vi "DecodeAvs47bReading.vi"(8 "LV ERROR IN":errorcluster, 10 "RXSTR":string="000000111001000000011000000000001100000010000000", 11 "CONFIGURATION CLUSTER":T1) -> (0 "LV ERROR OUT":errorcluster, 1 "ADC":i32, 2 "RESISTANCE":sgl format="%^#_6e", 3 "UNMODIFIED CONFIGURATION CLUSTER":T1, 4 "RESISTANCE STRING":string="0 ohm", 5 "ADC OVERRANGE":bool)   [LabVIEW 2023]
doc: "Used by ReadAvs47b.vi \nResistance given as real number"
panel:
  out "4 empty bits (hidden)":u16
  # "DecodeAvs47Reading.vi"
  # "(input to this VI)"
  # "(outputs)"
  # "(ohms)"
  # "Extracts the A/D conversion result from the Picobus return string RXSTR and \nexpresses the measured resistance as a floating point number. Also a string\nrepresentation with unit is provided for display purposes."
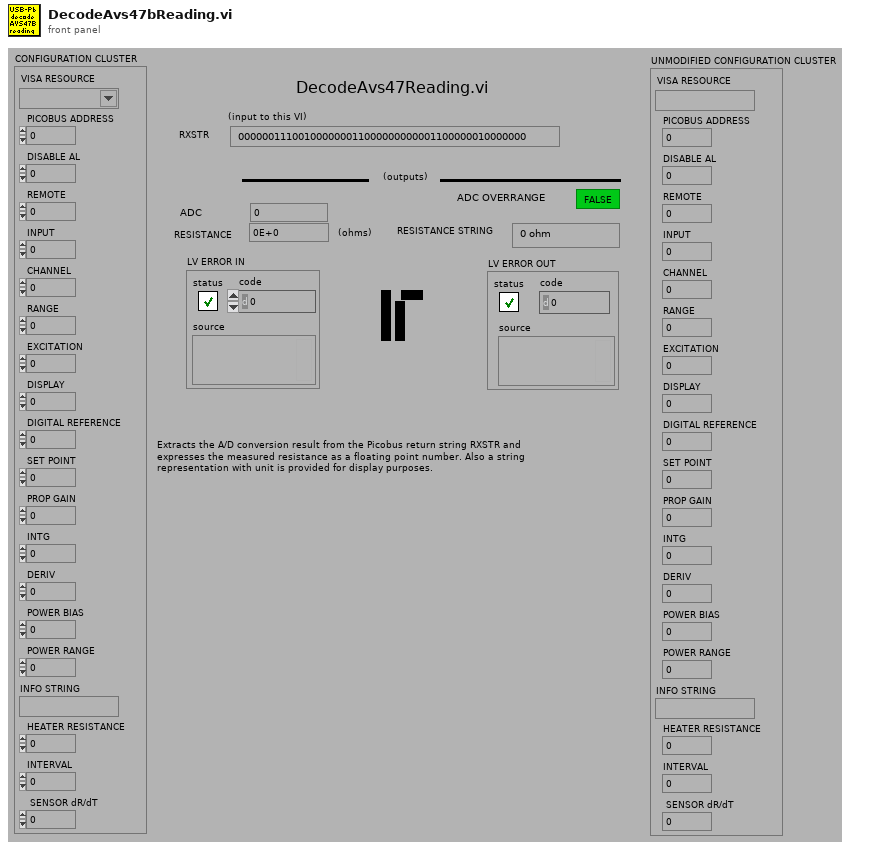
[diagram p1: front panel]
types:
  T1 = cluster{"VISA RESOURCE":refnum<visa-resource-name>, "PICOBUS ADDRESS":u8, "DISABLE AL":u8, "REMOTE":u8, "INPUT":u8, "CHANNEL":u8, "RANGE":u8, "EXCITATION":u8, "DISPLAY":u8, "DIGITAL REFERENCE":u16, "SET POINT":dbl, "PROP GAIN":u8, "INTG":u8, "DERIV":u8, "POWER BIAS":u8, "POWER RANGE":u8, "INFO STRING":string, "HEATER RESISTANCE":dbl, "INTERVAL":u8, " SENSOR dR/dT":u8}
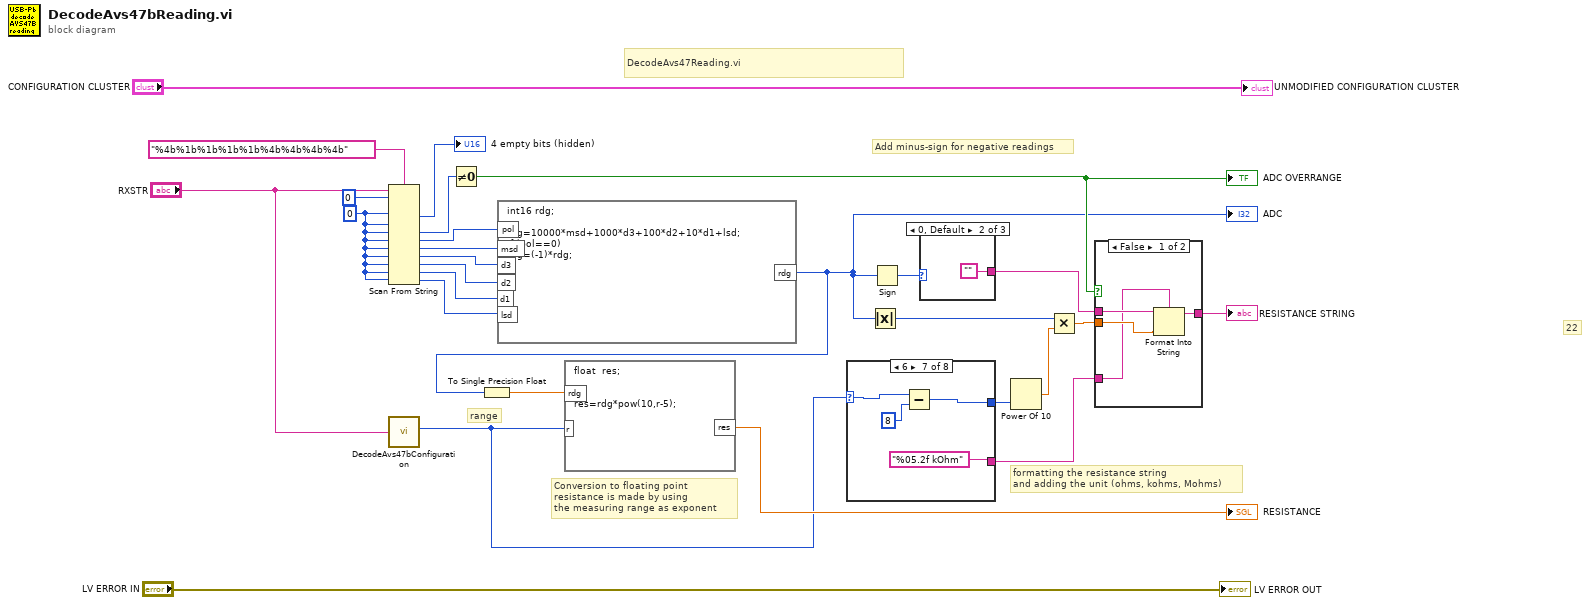
[diagram p0: block diagram]
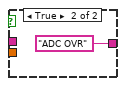
[diagram p2: hidden frame]
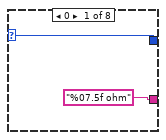
[diagram p3: hidden frame]
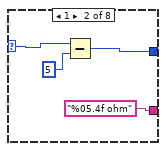
[diagram p4: hidden frame]
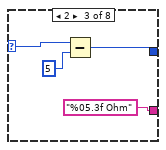
[diagram p5: hidden frame]
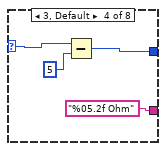
[diagram p6: hidden frame]
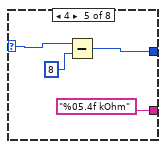
[diagram p7: hidden frame]
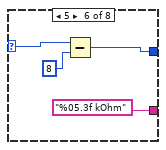
[diagram p8: hidden frame]
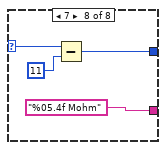
[diagram p9: hidden frame]
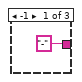
[diagram p10: hidden frame]
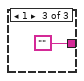
[diagram p11: hidden frame]
diagram:
  w24 = u16 0
  # "22"
  # "Add minus-sign for negative readings"
  # "formatting the resistance string\nand adding the unit (ohms, kohms, Mohms)"
  # "Conversion to floating point\nresistance is made by using \nthe measuring range as exponent"
  # "BCD-to-decimal\nconversion. Result\nis a 4 1/2 digit integer"
  # "range"
  # "DecodeAvs47Reading.vi"
  n1 = Scan From String(format string="%4b%1b%1b%1b%1b%4b%4b%4b%4b", input string="RXSTR", initial scan location=u16 0, default 1=w24, default 2=w24, default 3=w24, default 4=w24, default 5=w24, default 6=w24, default 7=w24, default 8=w24, default 9=w24) -> (output 1=→"4 empty bits (hidden)":u16, output 3=w14:u16, output 4=w18:u16, output 5=w23:u16, output 6=w22:u16, output 7=w21:u16, output 8=w20:u16, output 9=w19:u16)  [unwired: 2 in, 3 out]
  n2 = call "DecodeAvs47bConfiguration.vi"("RXSTR"="RXSTR") -> ("RANGE OUT"=w3:u16)  [unwired: 5 in, 4 out]
  n3 = Not Equal To 0?(x=w14) -> (x != 0?=w4:bool)
  "ADC OVERRANGE" <- w4
  n4 = formula code="int16 rdg;\n\nrdg=10000*msd+1000*d3+100*d2+10*d1+lsd;\nif (pol==0)\nrdg=(-1)*rdg;"("msd"=w23, "d3"=w22, "d2"=w21, "d1"=w20, "lsd"=w19, "pol"=w18) -> ("rdg"=w2:i16)
  "ADC" <- w2
  n5 = To Single Precision Float(number=w2) -> (single precision float=w16:sgl)
  n6 = formula code="float  res;\n\n\nres=rdg*pow(10,r-5);"("r"=w3, "rdg"=w16) -> ("res"=→"RESISTANCE":dbl)
  n7 = case shown="6" w3 {
    selector: w3 -> [w28 w31 w36 w39 w42 w46 w51 w55]
    tunnel: ["%07.5f ohm" "%05.4f ohm" ("format string") "%05.3f Ohm" ("format string") "%05.2f Ohm" ("format string") "%05.4f kOhm" ("format string") "%05.3f kOhm" ("format string") "%05.2f kOhm" ("format string") "%05.4f Mohm" ("format string")] -> w8
    tunnel: [w28 w30 w34 w38 w43 w47 w50 w54] -> w5
    frame 0 {
    }
    frame 1 {
      n8 = Subtract(x=w31, y=u8 5) -> (x-y=w30:u16)
    }
    frame 2 {
      n9 = Subtract(x=w36, y=u8 5) -> (x-y=w34:u16)
    }
    frame 3, Default {
      n10 = Subtract(x=w39, y=u8 5) -> (x-y=w38:u16)
    }
    frame 4 {
      n11 = Subtract(x=w42, y=u8 8) -> (x-y=w43:u16)
    }
    frame 5 {
      n12 = Subtract(x=w46, y=u8 8) -> (x-y=w47:u16)
    }
    frame 6 {
      n13 = Subtract(x=w51, y=u8 8) -> (x-y=w50:u16)
    }
    frame 7 {
      n14 = Subtract(x=w55, y=u8 11) -> (x-y=w54:u16)
    }
  }
  n15 = Absolute Value(x=w2) -> (abs(x)=w6:i16)
  n16 = Sign(1:w2) -> (0:w10:i16)
  n17 = case shown="0, Default" w10 {
    tunnel: ["-" "" ""] -> w9
    frame -1 {
    }
    frame 0, Default {
    }
    frame 1 {
    }
  }
  n18 = Power Of 10(x=w5) -> (10^x=w7:dbl)
  n19 = Multiply(x=w6, y=w7) -> (x*y=w11:dbl)
  n20 = case shown="False" w4 {
    tunnel: [w64 "ADC OVR"] -> w12
    tunnel: w11 -> [w63 _]
    tunnel: w9 -> [w62 _]
    tunnel: w8 -> [w61 _]
    frame False {
      n21 = Format Into String(format string=w61, initial string=w62, w63) -> (resulting string=w64:string)  [unwired: 1 in, 1 out]
    }
    frame True {
    }
  }
  "RESISTANCE STRING" <- w12
  "LV ERROR OUT" <- "LV ERROR IN"
  "UNMODIFIED CONFIGURATION CLUSTER" <- "CONFIGURATION CLUSTER"
